vi "h5_crtdat.vi"() -> ()   [LabVIEW 2009]
uses:
  Clients/H5F-File/H5F_ACC.ctl
panel:
  in  "filename":path
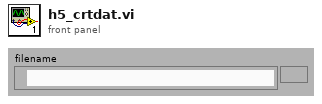
[diagram p1: front panel]
types:
  T1 = typedef "H5F_ACC.ctl" = enum16{"RDONLY", "RDWR", "TRUNC", "EXCL", "DEBUG", "CREAT"}
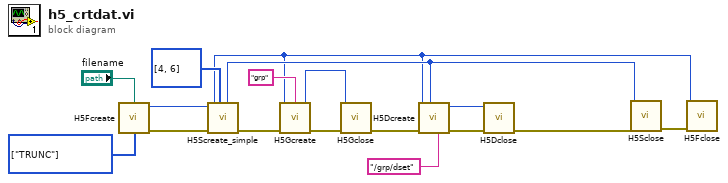
[diagram p0: block diagram]
diagram:
  w16 = T1[] [enum."TRUNC"] items=["RDONLY", "RDWR", "TRUNC", "EXCL", "DEBUG", "CREAT"] ("flags")
  n1 = call "H5Fcreate.vi"("filename"="filename", "flags"=w16) -> ("file_id"=w3:i32, "error out"=w15:errorcluster)  [unwired: 6 in]
  n2 = call "H5Screate_simple.vi"("dims"=u64[] [4, 6], "error in (no error)"=w15) -> ("error out"=w8:errorcluster, "space_id"=w11:i32)  [unwired: 7 in]
  n3 = call "H5Gcreate.vi"("name"="grp", "loc_id"=w3, "error in (no error)"=w8) -> ("group_id"=w6:i32, "error out"=w4:errorcluster)  [unwired: 5 in]
  n4 = call "H5Gclose.vi"("group_id"=w6, "error in (no error)"=w4) -> ("error out"=w2:errorcluster)  [unwired: 6 in, 1 out]
  n5 = call "H5Dcreate.vi"("file_id"=w3, "error in (no error)"=w2, "space_id"=w11, "name"="/grp/dset") -> ("dset_id"=w12:i32, "error out"=w5:errorcluster)  [unwired: 5 in]
  n6 = call "H5Dclose.vi"("error in (no error)"=w5, "dset_id"=w12) -> ("error out"=w1:errorcluster)  [unwired: 8 in, 1 out]
  n7 = call "H5Sclose.vi"("error in (no error)"=w1, "space_id"=w11) -> ("error out"=w9:errorcluster)  [unwired: 8 in, 1 out]
  n8 = call "H5Fclose.vi"("error in (no error)"=w9, "file_id"=w3) -> ()  [unwired: 8 in, 2 out]
